vi "Abnormal_Samples_Generator.vi"(10 "Sampling Info":T1, 11 "Number of Abnormal Samples":u32=1000) -> (3 "Abnormal Samples":sgl[][](array[numeric]))   [LabVIEW 2020]
uses:
  Controls/Sampling_Info.ctl
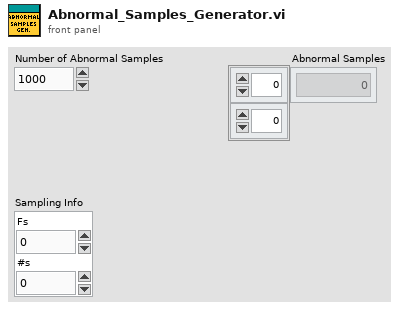
[diagram p1: front panel]
types:
  T1 = typedef "Sampling_Info.ctl" = cluster{"Fs":dbl, "#s":dbl}
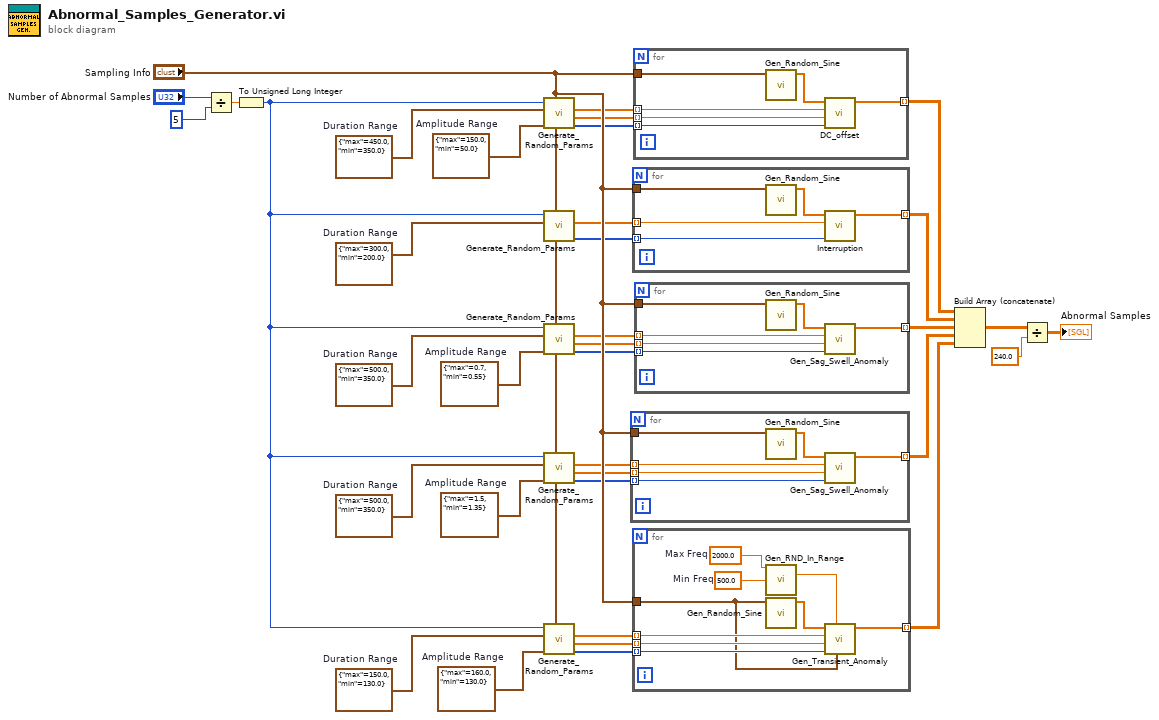
[diagram p0: block diagram]
diagram:
  w21 = cluster{"max":dbl, "min":dbl} {"max"=150.0, "min"=130.0}  # Duration Range
  w20 = cluster{"max":dbl, "min":dbl} {"max"=160.0, "min"=130.0}  # Amplitude Range
  w15 = cluster{"max":dbl, "min":dbl} {"max"=500.0, "min"=350.0}  # Duration Range
  w16 = cluster{"max":dbl, "min":dbl} {"max"=1.5, "min"=1.35}  # Amplitude Range
  w11 = cluster{"max":dbl, "min":dbl} {"max"=500.0, "min"=350.0}  # Duration Range
  w10 = cluster{"max":dbl, "min":dbl} {"max"=0.7, "min"=0.55}  # Amplitude Range
  w7 = cluster{"max":dbl, "min":dbl} {"max"=300.0, "min"=200.0}  # Duration Range
  w6 = cluster{"max":dbl, "min":dbl} {"max"=450.0, "min"=350.0}  # Duration Range
  w5 = cluster{"max":dbl, "min":dbl} {"max"=150.0, "min"=50.0}  # Amplitude Range
  n1 = Divide(x="Number of Abnormal Samples", y=5) -> (x/y=w31:dbl)
  n2 = To Unsigned Long Integer(number=w31) -> (unsigned 32bit integer=w35:u32)
  n3 = call "Generate_Random_Params.vi"("sampling info"="Sampling Info", "Amplitude Range"=w5, "Duration Range"=w6, "Dataset Samples"=w35) -> ("Duration"=w4:i32[], "Amplitude"=w3:sgl[], "Position"=w2:dbl[])  [unwired: 5 in]
  n4 = call "Generate_Random_Params.vi"("sampling info"="Sampling Info", "Duration Range"=w7, "Dataset Samples"=w35) -> ("Duration"=w9:i32[], "Position"=w8:dbl[])  [unwired: 6 in, 1 out]
  n5 = call "Generate_Random_Params.vi"("sampling info"="Sampling Info", "Amplitude Range"=w10, "Duration Range"=w11, "Dataset Samples"=w35) -> ("Duration"=w14:i32[], "Amplitude"=w13:sgl[], "Position"=w12:dbl[])  [unwired: 5 in]
  n6 = call "Generate_Random_Params.vi"("sampling info"="Sampling Info", "Amplitude Range"=w16, "Duration Range"=w15, "Dataset Samples"=w35) -> ("Duration"=w19:i32[], "Amplitude"=w18:sgl[], "Position"=w17:dbl[])  [unwired: 5 in]
  n7 = call "Generate_Random_Params.vi"("sampling info"="Sampling Info", "Amplitude Range"=w20, "Duration Range"=w21, "Dataset Samples"=w35) -> ("Duration"=w24:i32[], "Amplitude"=w23:sgl[], "Position"=w22:dbl[])  [unwired: 5 in]
  n8 = for {
    tunnel: [w41] -> w30 mode=indexing
    tunnel: w17 -> [w40] mode=indexing
    tunnel: w18 -> [w39] mode=indexing
    tunnel: w19 -> [w38] mode=indexing
    tunnel: "Sampling Info" -> [w37]
    n9 = call "Gen_Random_Sine.vi"("Sampling Info"=w37) -> ("data"=w42:sgl[])  [unwired: 10 in]
    n10 = call "Gen_Sag_Swell_Anomaly.vi"("Duration"=w38, "Amplitude"=w39, "Position"=w40, "Sine"=w42) -> ("Sine+Anomaly"=w41:sgl[])  [unwired: 7 in]
  }
  n11 = for {
    tunnel: [w47] -> w26 mode=indexing
    tunnel: w8 -> [w45] mode=indexing
    tunnel: w9 -> [w44] mode=indexing
    tunnel: "Sampling Info" -> [w43]
    n12 = call "Gen_Random_Sine.vi"("Sampling Info"=w43) -> ("data"=w46:sgl[])  [unwired: 10 in]
    n13 = call "Interruption.vi"("Duration"=w44, "Position"=w45, "Sine"=w46) -> ("Sine+Anomaly"=w47:sgl[])  [unwired: 8 in]
  }
  n14 = for {
    tunnel: [w55] -> w27 mode=indexing
    tunnel: w22 -> [w51] mode=indexing
    tunnel: w23 -> [w50] mode=indexing
    tunnel: w24 -> [w49] mode=indexing
    tunnel: "Sampling Info" -> [w48]
    w52 = 2000.0  # Max Freq
    w53 = 500.0  # Min Freq
    n15 = call "Gen_RND_In_Range.vi"("Upper Bound"=w52, "Lower Bound"=w53) -> ("RND_In_Range"=w54:dbl)  [unwired: 13 in]
    n16 = call "Gen_Random_Sine.vi"("Sampling Info"=w48) -> ("data"=w56:sgl[])  [unwired: 10 in]
    n17 = call "Gen_Transient_Anomaly.vi"("Sampling Info"=w48, "Frequency"=w54, "Tau"=w49, "Amplitude"=w50, "Position"=w51, "Sine"=w56) -> ("Sine+Anomaly"=w55:sgl[])  [unwired: 5 in]
  }
  n18 = for {
    tunnel: [w61] -> w25 mode=indexing
    tunnel: w2 -> [w60] mode=indexing
    tunnel: w3 -> [w59] mode=indexing
    tunnel: w4 -> [w58] mode=indexing
    tunnel: "Sampling Info" -> [w57]
    n19 = call "Gen_Random_Sine.vi"("Sampling Info"=w57) -> ("data"=w62:sgl[])  [unwired: 10 in]
    n20 = call "DC_offset.vi"("Duration"=w58, "Ampltude"=w59, "Position"=w60, "Sine"=w62) -> ("Sine+Anomaly"=w61:sgl[])  [unwired: 7 in]
  }
  n21 = for {
    tunnel: [w67] -> w28 mode=indexing
    tunnel: w12 -> [w66] mode=indexing
    tunnel: w13 -> [w65] mode=indexing
    tunnel: w14 -> [w64] mode=indexing
    tunnel: "Sampling Info" -> [w63]
    n22 = call "Gen_Random_Sine.vi"("Sampling Info"=w63) -> ("data"=w68:sgl[])  [unwired: 10 in]
    n23 = call "Gen_Sag_Swell_Anomaly.vi"("Duration"=w64, "Amplitude"=w65, "Position"=w66, "Sine"=w68) -> ("Sine+Anomaly"=w67:sgl[])  [unwired: 7 in]
  }
  n24 = Build Array (concatenate)(w25, w26, w28, w30, w27) -> (w29:sgl[][])
  n25 = Divide(x=w29, y=sgl 240.0) -> (x/y=→"Abnormal Samples":sgl[][])
